vi "Adjust TIS clock rate value.vi"(8 "error in (no error)":errorcluster, 11 "7976R_v1 in":refnum<class "7976R_v1.lvclass">) -> (0 "error out":errorcluster, 3 "7976R_v1 out":refnum<class "7976R_v1.lvclass">)   [LabVIEW 2015, in "7976R_v1.lvclass"]
uses:
  <userlib>/SE-APP-Receiver/NI5772/7976R_v1/7976R_v1.lvclass
  <userlib>/SE-APP-Receiver/NI5772/7976R_v1/7976R_v1.lvclass/7976R_v1.ctl
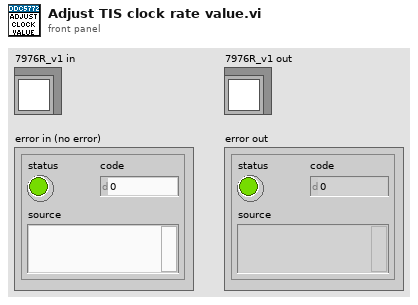
[diagram p1: front panel]
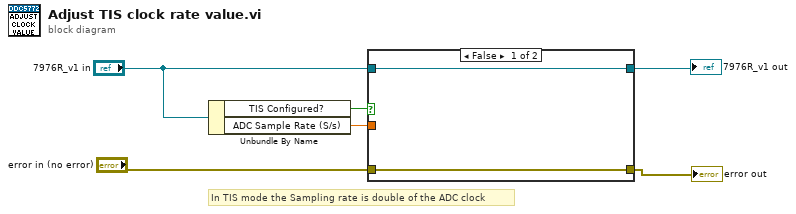
[diagram p0: block diagram]
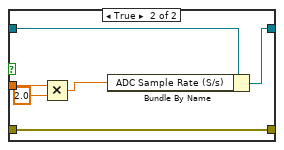
[diagram p2: hidden frame]
diagram:
  # "In TIS mode the Sampling rate is double of the ADC clock"
  n1 = Unbundle By Name("7976R_v1 in") -> ("TIS Configured?"=w3:bool, "ADC Sample Rate (S/s)"=w2:dbl)
  n2 = case shown="False" w3 {
    tunnel: "7976R_v1 in" -> [w8 w14]
    tunnel: w2 -> [_ w13]
    tunnel: [w8 w10] -> w4
    tunnel: "error in (no error)" -> [w7 w9]
    tunnel: [w7 w9] -> w6
    frame False {
    }
    frame True {
      n3 = Multiply(x=w13, y=2.0) -> (x*y=w11:dbl)
      n4 = Bundle By Name(cluster=w14, "ADC Sample Rate (S/s)"=w11) -> (w10:refnum<class "7976R_v1.lvclass">)
    }
  }
  "error out" <- w6
  "7976R_v1 out" <- w4
